vi "Read Data from  Waveform.vi"(8 "error in (no error)":errorcluster, 10 "Commands":string[](array[string])=["CALCulate:PN:DATA:XDATa?", "CALCulate:PN:TRAC:DATA:FDATa?"]) -> (0 "error out":errorcluster, 2 "Results":sgl[][](array[numeric]))   [LabVIEW 2017]
uses:
  <instrlib>/Agilent E5052X/Agilent E5052X.lvlib
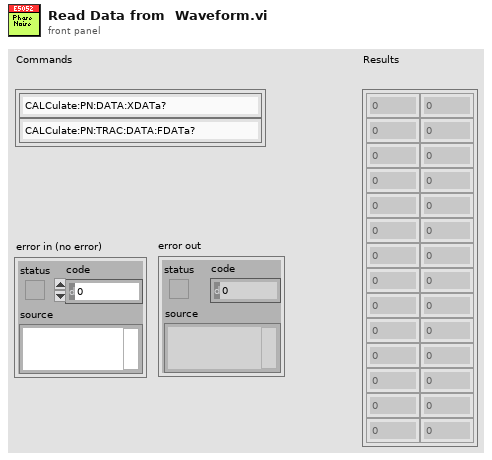
[diagram p1: front panel]
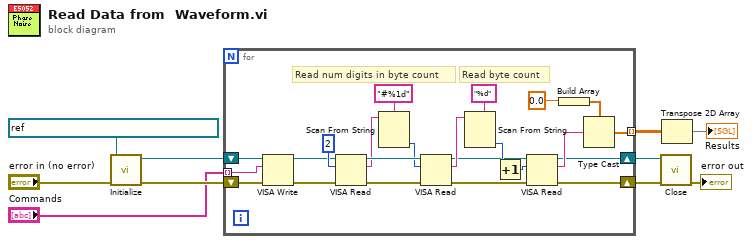
[diagram p0: block diagram]
diagram:
  n1 = call <instrlib>:"Initialize.vi"("error in (no error)"="error in (no error)", "VISA resource name"=refnum<visa-resource-name> "TCPIP0::192.168.1.100::inst0::INSTR") -> ("error out"=w6:errorcluster, "VISA resource name out"=w7:refnum<visa-resource-name>)  [unwired: 8 in]
  n2 = for {
    shift-right: [w17] -> w5
    shift-left: w7 -> [w33]
    shift-right: [w16] -> w4
    shift-left: w6 -> [w32]
    tunnel: "Commands" -> [w12] mode=indexing
    tunnel: [w11] -> w3 mode=indexing
    # "Read num digits in byte count"
    # "Read byte count"
    n3 = VISA Write(VISA resource name=w33, write buffer=w12, error in (no error)=w32) -> (VISA resource name out=w15:refnum<visa-resource-name>, error out=w14:errorcluster)  [unwired: 1 out]
    n4 = VISA Read(VISA resource name=w15, byte count=u32 2, error in (no error)=w14) -> (VISA resource name out=w28:refnum<visa-resource-name>, read buffer=w24:string, error out=w29:errorcluster)  [unwired: 1 out]
    n5 = Scan From String(format string="#%1d", input string=w24) -> (output 1=w27:i32)  [unwired: 3 in, 3 out]
    n6 = VISA Read(VISA resource name=w28, byte count=w27, error in (no error)=w29) -> (VISA resource name out=w22:refnum<visa-resource-name>, read buffer=w26:string, error out=w21:errorcluster)  [unwired: 1 out]
    n7 = Scan From String(format string="%d", input string=w26) -> (output 1=w23:i32)  [unwired: 3 in, 3 out]
    n8 = Increment(x=w23) -> (x+1=w13:i32)
    n9 = VISA Read(VISA resource name=w22, byte count=w13, error in (no error)=w21) -> (VISA resource name out=w17:refnum<visa-resource-name>, read buffer=w18:string, error out=w16:errorcluster)  [unwired: 1 out]
    n10 = Build Array(sgl 0.0) -> (w19:sgl[])
    n11 = Type Cast(type=w19, x=w18) -> (*(type *) &x=w11:sgl[])
  }
  n12 = call <instrlib>:"Close.vi"("error in (no error)"=w4, "VISA resource name"=w5) -> ("error out"=→"error out":errorcluster)  [unwired: 9 in]
  n13 = Transpose 2D Array(2D array=w3) -> (transposed array=→"Results":sgl[][])
